vi "2100_Test_Set State_Measure Resistance_Source and Sink_SP3T.vi"(0 "Semiconductor Module Context":T7, 1 "Script_Info":T3={"Script Name"="WalkingState", "All_Scripts"=[]}, 2 "current level":dbl=0.001 format="%#_13p", 3 "current range":dbl=0.001 format="%#_6p", 4 "Instrument_Pins":T6={"SMU_Pins"=["RF1", "RF2", "RF3", "RF4"], "HSDIO_Pins"=["CLK", "SDA"]}, 5 "Error In":errorcluster, 6 "USID":T4, 7 "Master_Register_Data_Array_In":T1 {"Address" format="%.0x"}, 10 "Publishable IDs":string[](array[string])=["State00", "State01", "State02", "State04", "State08"], 11 "Reg_Map_and_Bit_Name":T5={"Reg_Map_Bit_Name"="", "Reg_Map"=[["Reg Addr(0x00)", "7", "6", "5", "4", "3", "2", "1", "0"], ["0", "SPARE", "RF3_SH", "RF2_SH", "RF1_SH", "SPARE", "RF3_RFC", "RF2_RFC", "RF1_RFC"], ["1", "SPARE[7:0]", "", "", "", "", "", "", ""], ["2", "VVAR_EN", "LCM_EN", "RFC_SH", "SPARE", "VARACTOR[3:0]", "", "", ""], ["3", "SW_CTRL1_VIRTUAL[7:0]", "", "", "", "", "", "", ""], ["4", "SW_CTRL1_SWAP", "SW_CTRL1_RBSHIFT[2:0]", "", "", "SW_CTRL1_VSID[3:0]", "", "", ""], ["5", "REG_00_VIRTUAL_MASK[7:0]", "", "", "", "", "", "", ""], ["6", "LOCK_STATUS[1:0]", "", "CLK_DITHER", "FUSES_BURNED", "CLK_IDAC_CAL[3:0]", "", "", ""], ["7", "SPARE[2:0]", "", "", "ODFT_TRIM[4:0]", "", "", "", ""], ["8", "SPARE[2:0]", "", "", "HV_TRIM[4:0]", "", "", "", ""], ["9", "TEST_MUX[2:0]", "", "", "SPARE[1:0]", "", "MEMS_BG_TC[1:0]", "", "MEMSCP_RCM"], ["A", "CP_BOOST_OVRD_EN", "SPARE[2:0]", "", "", "PS_OFF_TIMER[1:0]", "", "PS_ON_TIMER[1:0]", ""], ["0", "", "", "", "", "", "", "", ""], ["D", "Reserved[1:0]", "", "WD_HI_EVENT_CNT[5:0]", "", "", "", "", ""], ["E", "VERSION_ID[7:0]", "", "", "", "", "", "", ""], ["F", "Reserved", "COUNT_200_LSB[6:0]", "", "", "", "", "", ""], ["10", "CLK_DIV2_EN", "Spare", "ODFT_EN", "HV_HYST[4:0]", "", "", "", ""], ["0", "", "", "", "", "", "", "", ""], ["12", "SHORT_FUSE", "FUSE_BURN", "STROBE_EN", "VIO_OK", "RTH[1:0]", "", "FUSE_LOAD_MAN_EN", "FUSE_LOAD"], ["13", "RR_ACK_EN", "Reserved", "ACK_POSITION[1:0]", "", "SuBUS_DRIVE_STRENGTH[3:0]", "", "", ""], ["14", "TM_IO_EN", "TM_IO_SEL", "SuBUS_OVS[1:0]", "", "Reserved[3:0]", "", "", ""], ["15", "Reserved[4:0]", "", "", "", "", "SuBUS_VERSION_PRESENT", "SuBUS_VOLTAGE", "SuBUS_FLAVOR_DEF"], ["16", "PROG_STROBE1_DUR[7:0]", "", "", "", "", "", "", ""], ["17", "PROG_STROBE0_DUR[7:0]", "", "", "", "", "", "", ""], ["18", "Reserved[2:0]", "", "", "EFUSE_SINGLE_ADDR_SEL[4:0]", "", "", "", ""], ["19", "POLL_ADR[4:0]", "", "", "", "", "POLL_BC[2:0]", "", ""], ["1A", "SOFTWARE_RESET", "Reserved[6:0]", "", "", "", "", "", ""], ["1B", "Reserved[7:0]", "", "", "", "", "", "", ""], ["1C", "PWR_MODE_1", "PWR_MODE_0", "TRIGGER_MASK[2:0]", "", "", "TRIGGER[2:0]", "", ""], ["1D", "PRODUCT_ID[7:0]", "", "", "", "", "", "", ""], ["1E", "MANUFACTURER_ID_LSB[7:0]", "", "", "", "", "", "", ""], ["1F", "MANUFACTURER_ID_MSB[3:0]", "", "", "", "USID[3:0]", "", "", ""]]}) -> (15 "Master_Register_Data_Array_Out":T1 {"Address" format="%.0x"}, 19 "Error Out":errorcluster)   [LabVIEW 2013]
uses:
  Controls/USID.ctl
  <vilib>/NI_TestStand_SemiconductorModule/NI_TestStand_Semiconductor_Module.lvlibp/PinMap/General/SemiconductorModuleContext.ctl
  Controls/Master_Reg_Data_Array.ctl
  Controls/Reg_Address_Data.ctl
  <vilib>/NI_TestStand_SemiconductorModule/NI_TestStand_Semiconductor_Module.lvlibp/PinMap/General/Publish/PublishDataDoubleFunctionalTest.vi
  <vilib>/NI_TestStand_SemiconductorModule/NI_TestStand_Semiconductor_Module.lvlibp
panel:
  out "Published_ID":string[](array[string])=["RF1", "RF2", "RF3", "RF4"]
  out "Data_to_LOG":dbl[](array[numeric]) format="%#_6p"
  in  "Tab Control":enum32{"Test Info", "Instrument Settings"}(tab)
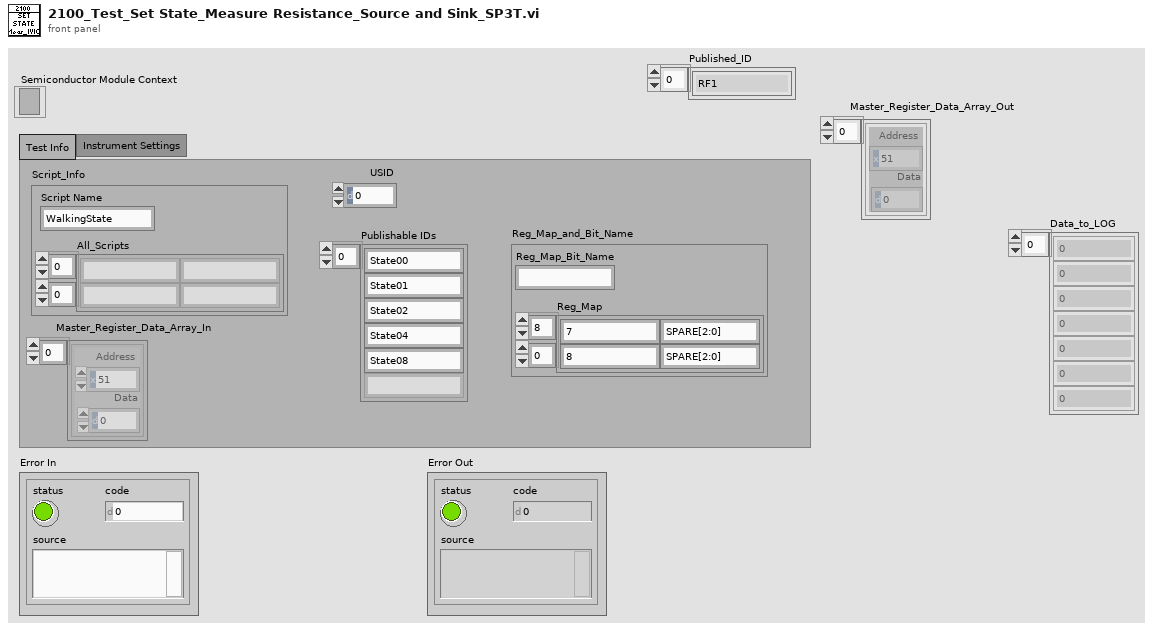
[diagram p1: front panel]
types:
  T1 = typedef "Master_Reg_Data_Array.ctl" = T2[]
  T2 = typedef "Reg_Address_Data.ctl" = cluster{"Address":u8, "Data":u8}
  T3 = cluster{"Script Name":string, "All_Scripts":string[][]}
  T4 = typedef "USID.ctl" = u8
  T5 = cluster{"Reg_Map_Bit_Name":string, "Reg_Map":string[][]}
  T6 = cluster{"SMU_Pins":string[], "HSDIO_Pins":string[]}
  T7 = typedef "NI_TestStand_Semiconductor_Module.lvlibp/SemiconductorModuleContext.ctl" = refnum<k7>
  T8 = typedef "Script Functions_Array.ctl" = enum16{"Reg_Write", "Bit_Write", "Delay", "Read", "Measure"}[]
  T9 = enum16{"Reg_Write", "Bit_Write", "Delay", "Read", "Measure"}
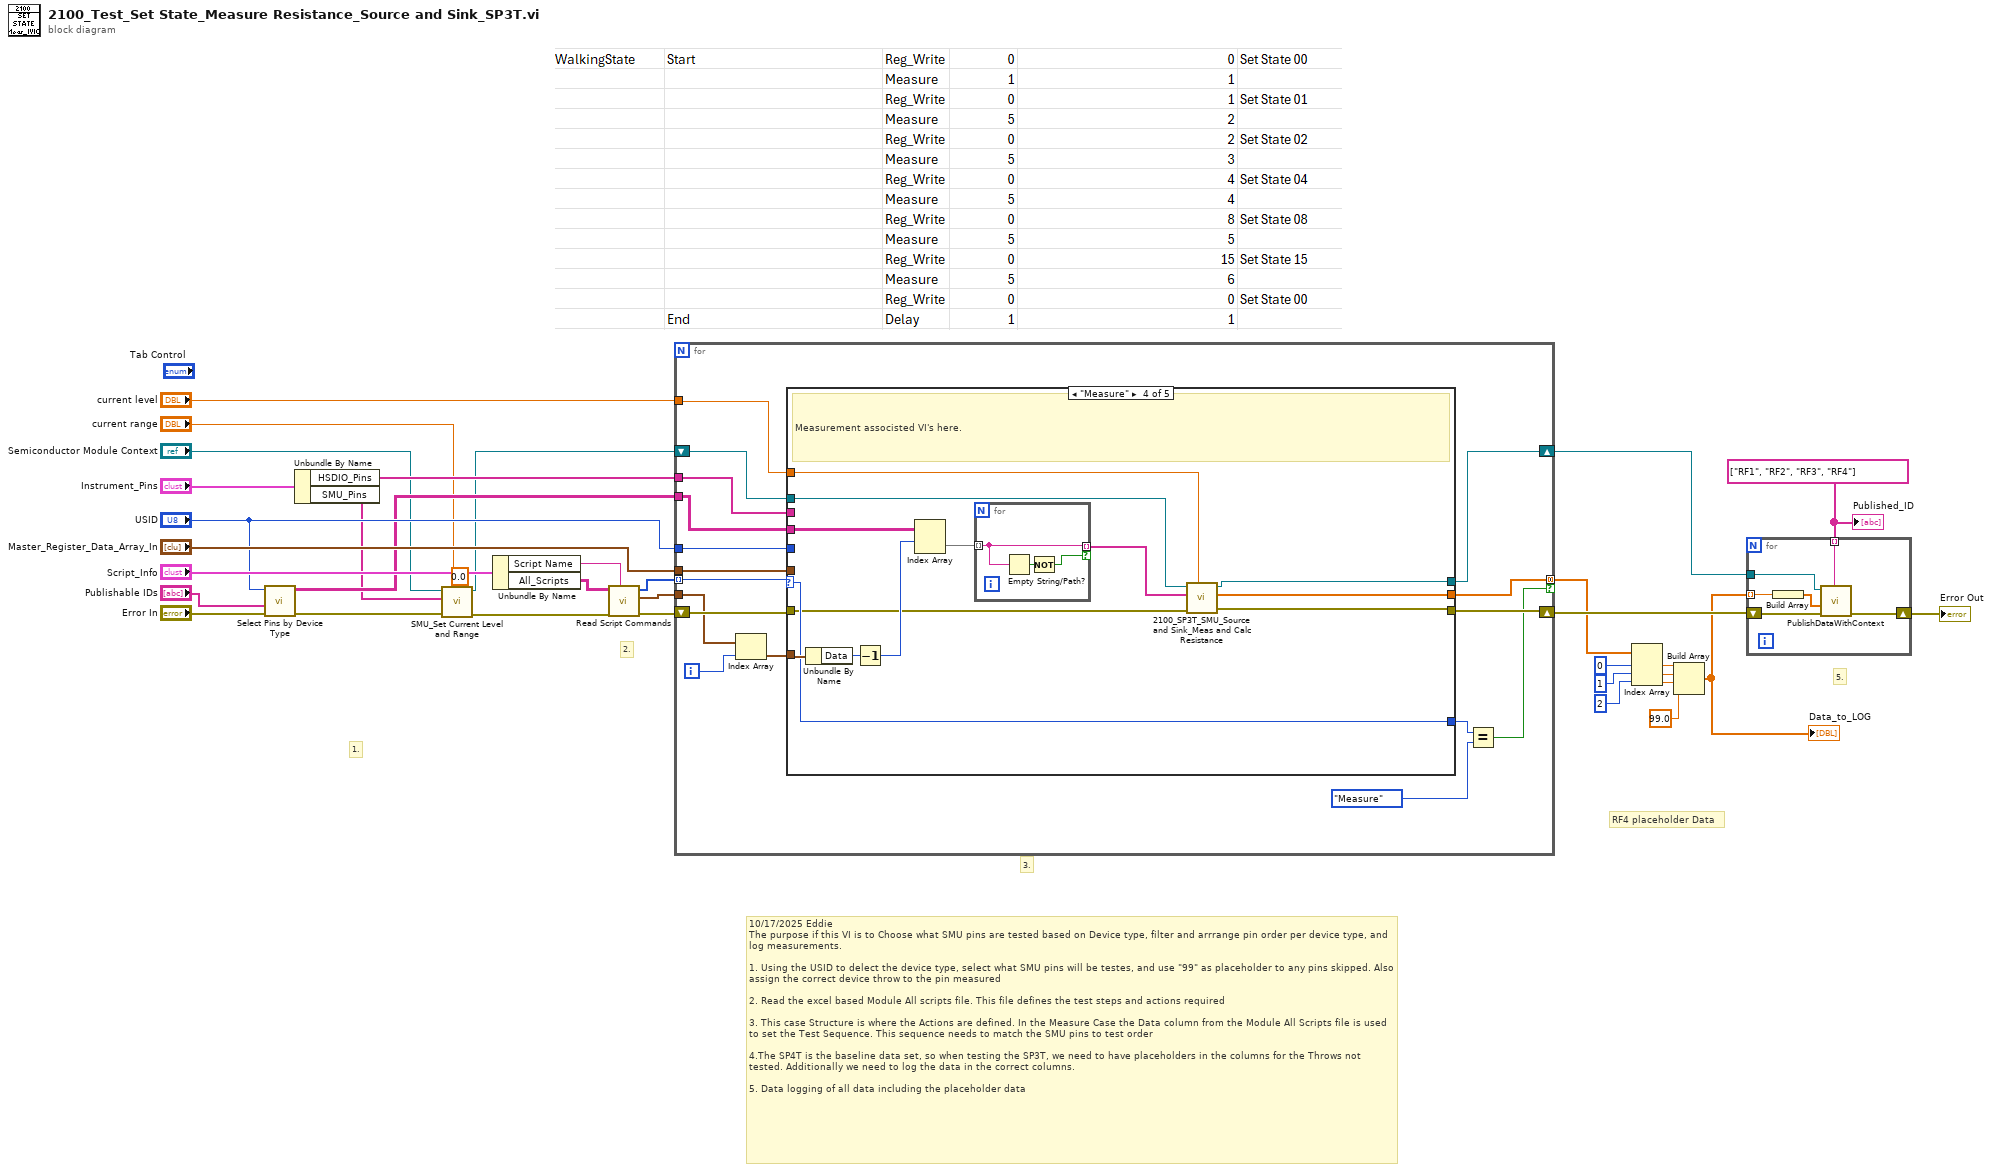
[diagram p0: block diagram]
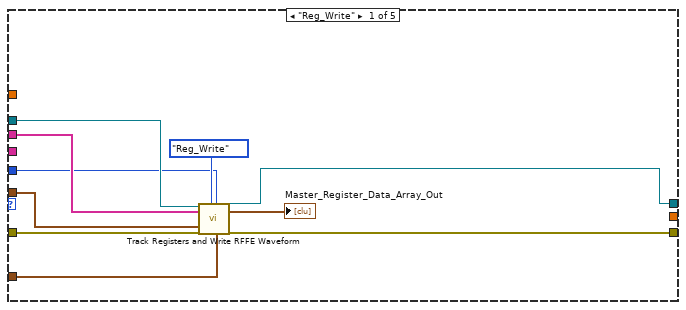
[diagram p2: hidden frame]
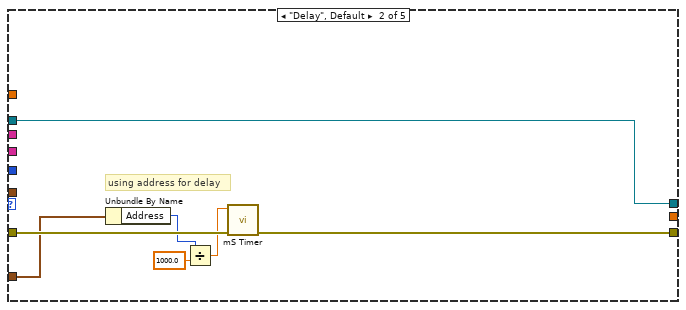
[diagram p3: hidden frame]
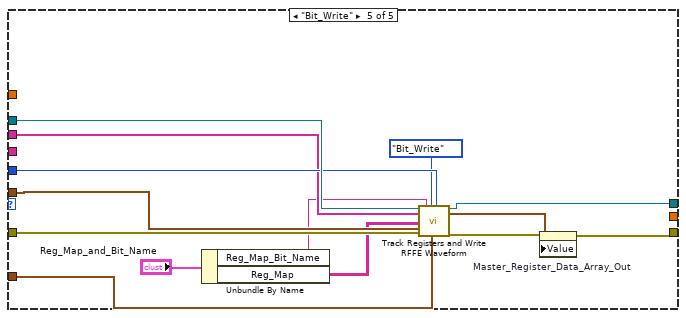
[diagram p5: hidden frame]
diagram:
  w19 = string[] ["RF1", "RF2", "RF3", "RF4"] ("SP4T_Pins")
  # "RF4 placeholder Data"
  # "10/17/2025 Eddie \nThe purpose if this VI is to Choose what SMU pins are tested based on Device type, filter and arrrange pin order per device type, and log measurements.\n\n1. Using the USID to delect the device type, select what SMU pins will be testes, and use \"99\" as placeholder to any pins skipped. Also assign the correct device throw to the pin measured\n\n2. Read the excel based Module All scripts file. This file defines the test steps and actions required\n\n3. This case Structure is where the Actions are defined. In the Measure Case the Data column from the Module All Scripts file is used to set the Test Sequence. This sequence needs to match the SMU pins to test order\n\n4.The SP4T is the baseline data set, so when testing the SP3T, we need to have placeholders in the columns for the Throws not tested. Additionally we need to log the data in the correct columns.\n\n5. Data logging of all data including the placeholder data"
  # "5."
  # "3."
  # "2."
  # "1."
  n1 = call "Select Pins by Device Type.vi"("error in (no error)"="Error In", "Publishable IDs_or Pins"="Publishable IDs", "USID"="USID") -> ("error out"=w18:errorcluster, "Pins to Test"=w23:string[][])  [unwired: 7 in]
  n2 = Unbundle By Name("Instrument_Pins") -> ("HSDIO_Pins"=w29:string[], "SMU_Pins"=w13:string[])
  n3 = call "SMU_Set Current Level and Range.vi"("current level"=0.0, "current range"="current range", "error in (no error)"=w18, "Pins"=w13, "Semiconductor Module Context"="Semiconductor Module Context") -> ("error out"=w17:errorcluster, "Semiconductor Module Context Out"=w14:T7)  [unwired: 5 in]
  n4 = Unbundle By Name("Script_Info") -> ("Script Name"=w26:string, "All_Scripts"=w27:string[][])
  n5 = call "Read Script Commands.vi"("Test Name"=w26, "Error In"=w17, "All_Scripts"=w27) -> ("Error Out"=w32:errorcluster, "Script_Data"=w33:T2[], "Script_Functions"=w34:T8)  [unwired: 5 in, 1 out]
  n6 = for {
    tunnel: "USID" -> [w45]
    tunnel: w34 -> [w44] mode=indexing
    tunnel: w33 -> [w48]
    tunnel: w29 -> [w49]
    shift-right: [w42] -> w20
    shift-left: w32 -> [w51]
    tunnel: "Master_Register_Data_Array_In" -> [w46]
    tunnel: w23 -> [w41]
    shift-right: [w40] -> w21
    shift-left: w14 -> [w50]
    tunnel: [w37] -> w9 mode=concatenating if=w36
    tunnel: "current level" -> [w35]
    i -> [w43]
    n7 = Index Array(array=w48, index=w43) -> (element=w47:T2)
    n8 = case shown="\"Measure\"" w44 {
      selector: w44 -> [_ _ _ w78 _]
      tunnel: w47 -> [w57 w67 _ w83 w87]
      tunnel: w51 -> [w61 w68 w70 w76 w100]
      tunnel: w45 -> [w54 _ _ _ w94]
      tunnel: w50 -> [w60 w62 w69 w75 w95]
      tunnel: w49 -> [w59 _ _ _ w92]
      tunnel: [w52 w66 w70 w74 w98] -> w42
      tunnel: w46 -> [w56 _ _ _ w91]
      tunnel: w41 -> [_ _ _ w82 _]
      tunnel: [w53 w62 w69 w77 w96] -> w40
      tunnel: [_ _ _ w78 _] -> w39
      tunnel: [_ _ _ w72 _] -> w37
      tunnel: w35 -> [_ _ _ w71 _]
      frame "Reg_Write" {
        n9 = call "Track Registers and Write RFFE Waveform.vi"("Semiconductor Module Context"=w60, "Pins"=w59, "Master_Register_Data_Array_In"=w56, "Error In"=w61, "Script_Functions"=enum16{"Reg_Write", "Bit_Write"}."Reg_Write", "USID"=w54, "Reg_Address_Data"=w57) -> ("Semiconductor Module Context Out"=w53:T7, "Master_Register_Data_Array_Out"=→"Master_Register_Data_Array_Out":T1, "Error Out"=w52:errorcluster)  [unwired: 10 in]
      }
      frame "Delay", Default {
        # "using address for delay"
        n10 = Unbundle By Name(w67) -> ("Address"=w64:u8)
        n11 = Divide(x=w64, y=1000.0) -> (x/y=w63:dbl)
        n12 = call "mS Timer.vi"("Error In"=w68, "Delay(S)"=w63) -> ("Error Out"=w66:errorcluster)  [unwired: 9 in]
      }
      frame "Read" {
        # "Future Dev Code"
      }
      frame "Measure" {
        # "Measurement associsted VI's here."
        n13 = Unbundle By Name(w83) -> ("Data"=w81:u8)
        n14 = Decrement(x=w81) -> (x-1=w79:u8)
        n15 = Index Array(array=w82, index (row)=w79) -> (element=w80:string[])  [unwired: 1 in]
        n16 = for {
          tunnel: w80 -> [w86] mode=indexing
          tunnel: [w86] -> w73 mode=indexing if=w84
          n17 = Empty String/Path?(string/path=w86) -> (empty?=w85:bool)
          n18 = Not(x=w85) -> (.not. x?=w84:bool)
        }
        n19 = call "2100_SP3T_SMU_Source and Sink_Meas and Calc Resistance.vi"("Current  Level"=w71, "error in (no error)"=w76, "Pins"=w73, "Semiconductor Module Context"=w75) -> ("error Out"=w74:errorcluster, "Avg_Individual_Throws"=w72:dbl[], "Semiconductor Module Context Out"=w77:T7)  [unwired: 4 in, 1 out]
      }
      frame "Bit_Write" {
        n20 = Unbundle By Name("Reg_Map_and_Bit_Name") -> ("Reg_Map_Bit_Name"=w89:string, "Reg_Map"=w88:string[][])
        n21 = call "Track Registers and Write RFFE Waveform.vi"("Semiconductor Module Context"=w95, "Pins"=w92, "Reg_Map"=w88, "Master_Register_Data_Array_In"=w91, "Error In"=w100, "Reg_Map_Bit_Name"=w89, "Script_Functions"=enum16{"Reg_Write", "Bit_Write"}."Bit_Write", "USID"=w94, "Reg_Address_Data"=w87) -> ("Semiconductor Module Context Out"=w96:T7, "Master_Register_Data_Array_Out"=w97:T1, "Error Out"=w99:errorcluster)  [unwired: 8 in]
        n22 = property on="Master_Register_Data_Array_Out" class="Arr (strict)"(error in=w99, "Value"=w97) -> (error out=w98:errorcluster)  [unwired: 1 in, 1 out]
      }
    }
    n23 = Equal?(x=w39, y=T9."Measure" ("Enum")) -> (x = y?=w36:bool)
  }
  n24 = Index Array(array=w9, index #1=0 ("index"), index #2=1 ("index"), index #3=2 ("index")) -> (element #1=w5:dbl, element #2=w4:dbl, element #3=w3:dbl)
  n25 = Build Array(w5, w4, w3, 99.0 ("element")) -> (w1:dbl[])
  "Data_to_LOG" <- w1
  n26 = for {
    shift-right: [w106] -> w22
    shift-left: w20 -> [w105]
    tunnel: w21 -> [w104]
    tunnel: w19 -> [w103] mode=indexing
    tunnel: w1 -> [w101] mode=indexing
    n27 = Build Array(w101) -> (w102:dbl[])
    n28 = call-poly <vilib>:"PublishDataWithContext.vi"("Published Data Id"=w103, "error in (no error)"=w105, "Data In"=w102, "Semiconductor Module Context"=w104) -> ("error out"=w106:errorcluster)  [unwired: 6 in, 1 out]
  }
  "Error Out" <- w22
  "Published_ID" <- w19
